vi "Initialize (Physical Channel).vi"(0 "physical channels":refnum<k21>, 7 "reservation access (Read/Write)":i32(ring)=3 items=["None"=0, "Read Only"=1, "Read/Write"=3], 9 "reservation group":string, 11 "error in (no error)":errorcluster, 12 "connect timeout (60 sec)":dbl=60.0) -> (4 "SLSC Local out":refnum<class "SLSC Local.lvclass">, 15 "error out":errorcluster)   [LabVIEW 2015, in "SLSC Local.lvclass"]
uses:
  SLSC Local.lvclass
  SLSC Local.lvclass/SLSC Local.ctl
  <vilib>/SLSC/Initialize Session with Phys Chans.vi
  <vilib>/SLSC/SLSC.lvlib
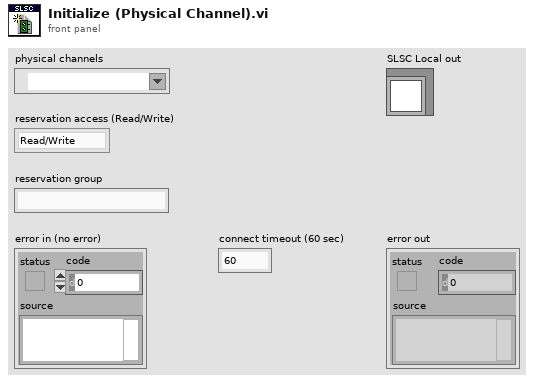
[diagram p1: front panel]
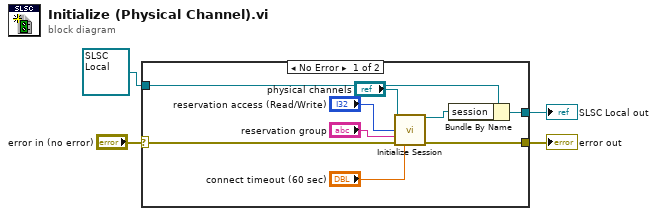
[diagram p0: block diagram]
diagram:
  n1 = case shown="No Error" "error in (no error)" {
    selector: "error in (no error)" -> [w11 w15]
    tunnel: [w10 w15] -> w3
    tunnel: [w12 w14] -> w1
    tunnel: refnum<class "SLSC Local.lvclass"> refnum ("SLSC Local in") -> [w13 w14]
    frame No Error {
      n2 = call-poly <vilib>:"Initialize Session.vi"("physical channels"="physical channels", "reservation access (Read/Write)"="reservation access (Read/Write)", "reservation group"="reservation group", "error in (no error)"=w11, "connect timeout (60 sec)"="connect timeout (60 sec)") -> ("session out"=w9:refnum<k21>, "error out"=w10:errorcluster)  [unwired: 9 in]
      n3 = Bundle By Name(cluster=w13, "session"=w9) -> (w12:refnum<class "SLSC Local.lvclass">)
    }
    frame Error {
    }
  }
  "error out" <- w3
  "SLSC Local out" <- w1
